vi "Max Spin Range Test.vi"(8 "Error In":errorcluster, 9 "lower limit":i32, 10 "upper limit":i32, 11 "GEA2 Reference In":refnum<k24>) -> (0 "Error Out":errorcluster, 1 "Pass/Fail?":bool, 2 "Report Text":string, 3 "GEA2 Reference Out":refnum<k24>)   [LabVIEW 2016]
doc: "This VI reads ERD 2032 and tests that it is within specified bounds."
uses:
  Q:/Common/DLLs/GEA3/GeaCommunication.dll
  Common/DLLs/GEA3/GeaCommunication.dll
  Common/LabVIEW GEA2 Toolkit/LabVIEW_GEA2_Toolkit.lvlibp/type defs/Source_Destination.ctl
  Common/LabVIEW GEA2 Toolkit/LabVIEW_GEA2_Toolkit.lvlibp/type defs/ERD Read Data In.ctl
  Common/LabVIEW GEA2 Toolkit/LabVIEW_GEA2_Toolkit.lvlibp/type defs/Data Type.ctl
  Common/LabVIEW GEA2 Toolkit/LabVIEW_GEA2_Toolkit.lvlibp
panel:
  in  "GEA Inputs":T1={"Source"=228, "Destination"=35} {"Destination" format="%.0x"; "Source" format="%.0x"}
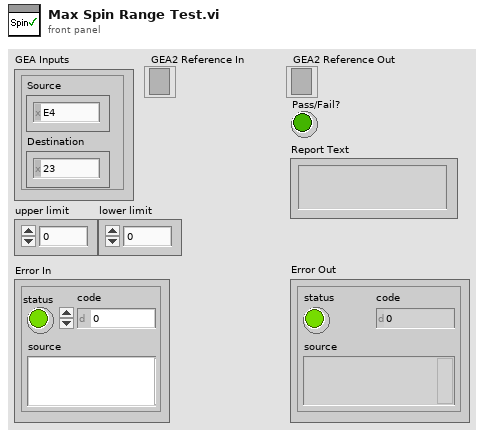
[diagram p1: front panel]
types:
  T1 = typedef "LabVIEW_GEA2_Toolkit.lvlibp/Source_Destination.ctl" = cluster{"Source":u8, "Destination":u8}
  T2 = typedef "LabVIEW_GEA2_Toolkit.lvlibp/ERD Read Data In.ctl" = cluster{"ERD Number":u16, "Data Type":T3}
  T3 = typedef "LabVIEW_GEA2_Toolkit.lvlibp/Data Type.ctl" = enum16{"string", "boolean", "uint8_t", "uint16_t", "uint32_t", "uint64_t", "int8_t", "int16_t", "int32_t", "int64_t"}
  T4 = typedef "LabVIEW_GEA2_Toolkit.lvlibp/ERD Read Data Out.ctl" = cluster{"ERD Number":u16, "Data":string}
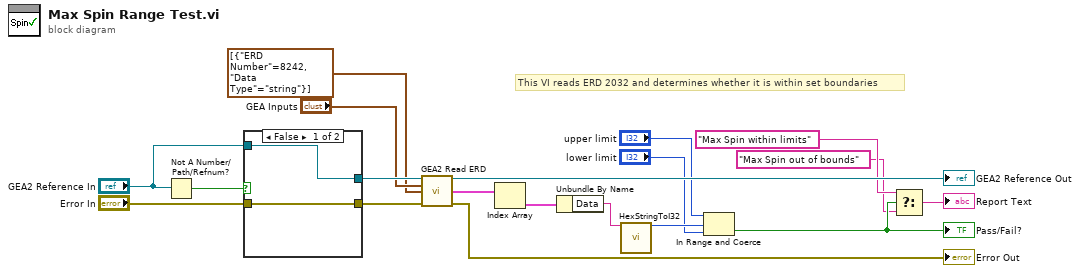
[diagram p0: block diagram]
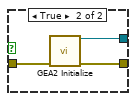
[diagram p2: hidden frame]
diagram:
  # "This VI reads ERD 2032 and determines whether it is within set boundaries"
  n1 = Not A Number/Path/Refnum?(number/path/refnum="GEA2 Reference In") -> (NaN/Path/Refnum?=w17:bool)
  n2 = case shown="False" w17 {
    tunnel: [w21 w24] -> w16
    tunnel: "GEA2 Reference In" -> [w21 _]
    tunnel: "Error In" -> [w20 w23]
    tunnel: [w20 w22] -> w15
    frame False {
    }
    frame True {
      n3 = call "GEA2 Initialize.vi"("error in"=w23) -> ("GEA2 Reference Out"=w24:refnum<k24>, "error out"=w22:errorcluster)  [unwired: 12 in, 1 out]
    }
  }
  n4 = call "GEA2 Read ERD.vi"("GEA2 Reference In"=w16, "GEA Inputs"="GEA Inputs", "Read ERD List"=T2[] [{"ERD Number"=8242, "Data Type"=enum."string"}], "Error In"=w15) -> ("GEA2 Reference Out"=→"GEA2 Reference Out":refnum<k24>, "ERD Data Out"=w12:T4[], "Error Out"=→"Error Out":errorcluster)  [unwired: 8 in, 1 out]
  n5 = Index Array(array=w12) -> (element=w11:T4)  [unwired: 1 in]
  n6 = Unbundle By Name(w11) -> ("Data"=w10:string)
  n7 = call "HexStringToI32.vi"("Input String"=w10) -> ("Number Out"=w9:i32)  [unwired: 14 in]
  n8 = In Range and Coerce(upper limit="upper limit", x=w9, lower limit="lower limit") -> (In Range?=w4:bool)  [unwired: 1 out]
  "Pass/Fail?" <- w4
  n9 = Select(t="Max Spin within limits", s=w4, f="Max Spin out of bounds") -> (s? t:f=→"Report Text":string)
